vi "Plot Test (Scope Screen 3).vi"() -> ()   [LabVIEW 2021]
uses:
  <vilib>/measure/NI_MABase.lvlib
panel:
  in  "Cursor.Cursor Plot":i32
  in  "Y Scale.Range:Minimum":dbl
  in  "Y Scale.Range:Maximum":dbl
  in  "Active Y Scale":i32
  in  "Plot.Visible":bool
  in  "Active Plot":u32
  in  "Cursor.Cursor Position:Cursor X":dbl
  in  "Active Cursor":u32
  in  "amplitude 2":dbl=1.0 format="%0.2p"
  in  "frequency 2":dbl=10.0 format="%0.2p"
  in  "amplitude":dbl=1.0 format="%0.2p"
  in  "frequency":dbl=10.0 format="%0.2p"
  in  "stop":bool
  out "Waveform Graph":waveform(dbl)[](graph)
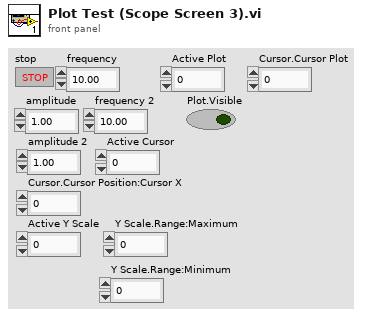
[diagram p1: front panel]
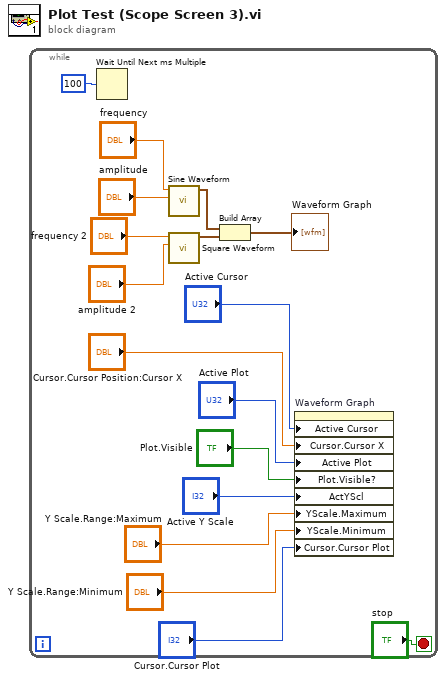
[diagram p0: block diagram]
diagram:
  n1 = while {
    stop <- "stop" stop-if-true
    n2 = Wait Until Next ms Multiple(millisecond multiple=u32 100) -> ()  [unwired: 1 out]
    n3 = call <vilib>:"Sine Waveform.vi"("amplitude"="amplitude", "frequency"="frequency") -> ("signal out"=w11:waveform(dbl))  [unwired: 8 in, 1 out]
    n4 = call <vilib>:"Square Waveform.vi"("amplitude"="amplitude 2", "frequency"="frequency 2") -> ("signal out"=w10:waveform(dbl))  [unwired: 8 in, 1 out]
    n5 = Build Array(w11, w10) -> (→"Waveform Graph":waveform(dbl)[])
    n6 = property on="Waveform Graph" class="WFGraph (strict)"("Active Cursor"="Active Cursor", "Cursor.Cursor X"="Cursor.Cursor Position:Cursor X", "Active Plot"="Active Plot", "Plot.Visible?"="Plot.Visible", "ActYScl"="Active Y Scale", "YScale.Maximum"="Y Scale.Range:Maximum", "YScale.Minimum"="Y Scale.Range:Minimum", "Cursor.Cursor Plot"="Cursor.Cursor Plot") -> ()  [unwired: 2 in, 2 out]
  }
